vi "Initialize.vi"(8 "error in (no error)":errorcluster, 11 "GW-SpitOut-Cmd in":refnum<class "GW-SpitOut-Cmd.lvclass">) -> (0 "error out":errorcluster, 3 "GW-SpitOut-Cmd out":refnum<class "GW-SpitOut-Cmd.lvclass">)   [LabVIEW 2013, in "GW-SpitOut-Cmd.lvclass"]
uses:
  GW-SpitOut-Cmd.lvclass
  States/GW-SpittingOut-State/GW-SpittingOut-State.lvclass
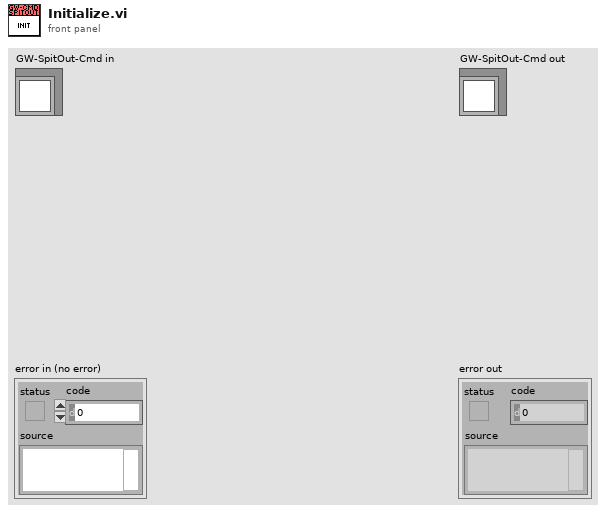
[diagram p1: front panel]
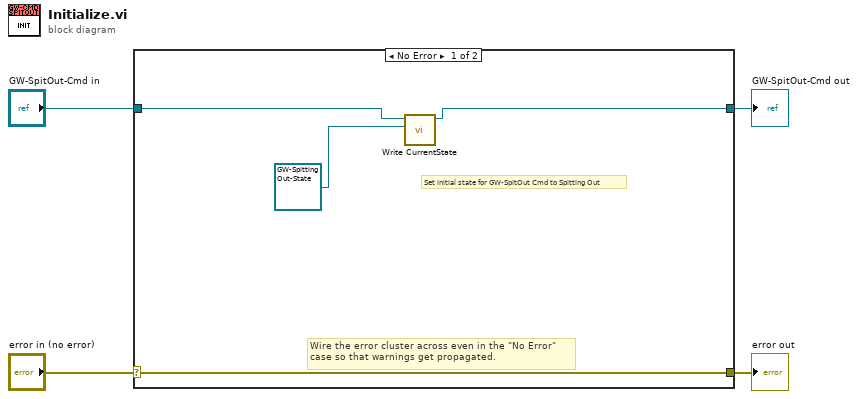
[diagram p0: block diagram]
diagram:
  n1 = case shown="No Error" "error in (no error)" {
    selector: "error in (no error)" -> [w8 w10]
    tunnel: [w8 w10] -> w3
    tunnel: [w6 w9] -> w1
    tunnel: "GW-SpitOut-Cmd in" -> [w7 w9]
    frame No Error {
      # "Set initial state for GW-SpitOut Cmd to Spitting Out"
      # "Wire the error cluster across even in the \"No Error\"\ncase so that warnings get propagated."
      n2 = call-dynamic "Write CurrentState.vi"("State.lvclass"=refnum<class "GW-SpittingOut-State.lvclass"> refnum ("GW-SpittingOut-State.lvclass"), "Command in"=w7) -> ("Command out"=w6:refnum<class "GW-SpitOut-Cmd.lvclass">)  [unwired: 8 in, 1 out]
    }
    frame Error {
    }
  }
  "error out" <- w3
  "GW-SpitOut-Cmd out" <- w1
